vi "HFRR ADV v01.vi"() -> ()   [LabVIEW 2023] (continued)
1.5095757095675688, 1.5106502499343546, 1.5103432384009872, 1.5104967441676709, 1.5111107672344057, 1.5104967441676709, 1.5103432384009872, 1.5112642730010895, 1.5108037557010383, 1.5103432384009872, 1.5104967441676709, 1.5106502499343546, 1.5106502499343546, 1.5108037557010383, 1.5111107672344057, 1.5095757095675688, 1.5097292153342525, 1.5111107672344057, 1.5104967441676709, 1.5138738710347124, 1.5138738710347124, 1.5124923191345592, 1.5115712845344569, 1.510957261467722, 1.509422203800885, 1.5108037557010383, 1.5104967441676709, 1.5101897326343034, 1.5104967441676709, 1.5101897326343034, 1.5101897326343034, 1.5103432384009872, 1.5101897326343034, 1.5104967441676709, 1.5101897326343034, 1.5108037557010383, 1.5106502499343546, 1.5098827211009362, 1.5112642730010895, 1.5098827211009362, 1.510957261467722, 1.5104967441676709, 1.5101897326343034, 1.5101897326343034, 1.5103432384009872, 1.5108037557010383, 1.5097292153342525, 1.5111107672344057, 1.5108037557010383, 1.5104967441676709, 1.5112642730010895, 1.5103432384009872, 1.5097292153342525, 1.5104967441676709, 1.5106502499343546, 1.5108037557010383, 1.5100362268676197, 1.5106502499343546, 1.5106502499343546, 1.5103432384009872, 1.5097292153342525, 1.5106502499343546, 1.5100362268676197, 1.5111107672344057, 1.5108037557010383, 1.5100362268676197, 1.5101897326343034, 1.5117247903011406, 1.5117247903011406, 1.510957261467722, 1.5100362268676197, 1.510957261467722, 1.5112642730010895, 1.5103432384009872, 1.5112642730010895, 1.5098827211009362, 1.5112642730010895, 1.510957261467722, 1.5106502499343546, 1.5123388133678755, 1.5123388133678755, 1.5103432384009872, 1.5101897326343034, 1.5101897326343034, 1.5104967441676709, 1.5097292153342525, 1.5111107672344057, 1.5108037557010383, 1.5126458249012429, 1.5117247903011406, 1.5100362268676197, 1.5106502499343546, 1.5098827211009362, 1.5104967441676709, 1.5098827211009362, 1.5106502499343546, 1.5115712845344569, 1.5108037557010383, 1.5112642730010895, 1.5100362268676197, 1.5112642730010895, 1.5104967441676709, 1.5098827211009362, 1.5091151922675177, 1.5112642730010895, 1.5103432384009872, 1.514641399868131, 1.5154089287015495, 1.5117247903011406, 1.5111107672344057, 1.5101897326343034, 1.5098827211009362, 1.5106502499343546, 1.5106502499343546, 1.5106502499343546, 1.5106502499343546, 1.5104967441676709, 1.5112642730010895, 1.5103432384009872, 1.5108037557010383, 1.5106502499343546, 1.5097292153342525, 1.510957261467722, 1.5112642730010895, 1.5103432384009872, 1.510957261467722, 1.5112642730010895, 1.5111107672344057, 1.5106502499343546, 1.5097292153342525, 1.5101897326343034, 1.5097292153342525, 1.5114177787677732, 1.5100362268676197, 1.5103432384009872, 1.5114177787677732, 1.5104967441676709, 1.5112642730010895, 1.5108037557010383, 1.509422203800885, 1.5108037557010383, 1.510957261467722, 1.5108037557010383, 1.5108037557010383, 1.5106502499343546, 1.5108037557010383, 1.510957261467722, 1.5117247903011406, 1.5092686980342014, 1.5098827211009362, 1.5108037557010383, 1.5104967441676709, 1.510957261467722, 1.5111107672344057, 1.5114177787677732, 1.5114177787677732, 1.5114177787677732, 1.5100362268676197, 1.509422203800885, 1.5114177787677732, 1.5106502499343546, 1.5100362268676197, 1.5108037557010383, 1.5103432384009872, 1.5108037557010383, 1.510957261467722, 1.5101897326343034, 1.5103432384009872, 1.5098827211009362, 1.5114177787677732, 1.5108037557010383, 1.5104967441676709, 1.510957261467722, 1.5101897326343034, 1.5111107672344057, 1.5106502499343546, 1.5103432384009872, 1.5108037557010383, 1.5095757095675688, 1.5106502499343546, 1.5103432384009872, 1.5104967441676709, 1.5111107672344057, 1.5104967441676709, 1.5103432384009872, 1.5112642730010895, 1.5108037557010383, 1.5103432384009872, 1.5104967441676709, 1.5106502499343546, 1.5106502499343546, 1.5108037557010383, 1.5111107672344057, 1.5095757095675688, 1.5097292153342525, 1.5111107672344057, 1.5104967441676709, 1.5138738710347124, 1.5138738710347124, 1.5124923191345592, 1.5115712845344569, 1.510957261467722, 1.509422203800885, 1.5108037557010383, 1.5104967441676709, 1.5101897326343034, 1.5104967441676709, 1.5101897326343034, 1.5101897326343034, 1.5103432384009872, 1.5101897326343034, 1.5104967441676709, 1.5101897326343034, 1.5108037557010383, 1.5106502499343546, 1.5098827211009362, 1.5112642730010895, 1.5098827211009362, 1.510957261467722, 1.5104967441676709, 1.5101897326343034, 1.5101897326343034, 1.5103432384009872, 1.5108037557010383, 1.5097292153342525, 1.5111107672344057, 1.5108037557010383, 1.5104967441676709, 1.5112642730010895, 1.5103432384009872, 1.5097292153342525, 1.5104967441676709, 1.5106502499343546, 1.5108037557010383, 1.5100362268676197, 1.5106502499343546, 1.5106502499343546, 1.5103432384009872, 1.5097292153342525, 1.5106502499343546, 1.5100362268676197, 1.5111107672344057, 1.5108037557010383, 1.5100362268676197, 1.5101897326343034, 1.5117247903011406, 1.5117247903011406, 1.510957261467722, 1.5100362268676197, 1.510957261467722, 1.5112642730010895, 1.5103432384009872, 1.5112642730010895, 1.5098827211009362, 1.5112642730010895, 1.510957261467722, 1.5106502499343546, 1.5123388133678755, 1.5123388133678755, 1.5103432384009872, 1.5101897326343034, 1.5101897326343034, 1.5104967441676709, 1.5097292153342525, 1.5111107672344057, 1.5108037557010383, 1.5126458249012429, 1.5117247903011406, 1.5100362268676197, 1.5106502499343546, 1.5098827211009362, 1.5104967441676709, 1.5098827211009362, 1.5106502499343546, 1.5115712845344569, 1.5108037557010383, 1.5112642730010895, 1.5100362268676197, 1.5112642730010895, 1.5104967441676709, 1.5098827211009362, 1.5091151922675177, 1.5112642730010895, 1.5103432384009872, 1.514641399868131, 1.5154089287015495, 1.5117247903011406, 1.5111107672344057, 1.5101897326343034, 1.5098827211009362, 1.5106502499343546, 1.5106502499343546, 1.5106502499343546, 1.5106502499343546, 1.5104967441676709, 1.5112642730010895, 1.5103432384009872, 1.5108037557010383, 1.5106502499343546, 1.5097292153342525, 1.510957261467722, 1.5112642730010895, 1.5103432384009872, 1.510957261467722, 1.5112642730010895, 1.5111107672344057, 1.5106502499343546, 1.5097292153342525, 1.5101897326343034, 1.5097292153342525, 1.5114177787677732, 1.5100362268676197, 1.5103432384009872, 1.5114177787677732, 1.5104967441676709, 1.5112642730010895, 1.5108037557010383, 1.509422203800885, 1.5108037557010383, 1.510957261467722, 1.5108037557010383, 1.5108037557010383, 1.5106502499343546, 1.5108037557010383, 1.510957261467722, 1.5117247903011406, 1.5092686980342014, 1.5098827211009362, 1.5108037557010383, 1.5104967441676709, 1.510957261467722, 1.5111107672344057, 1.5114177787677732, 1.5114177787677732, 1.5114177787677732, 1.5100362268676197, 1.509422203800885, 1.5114177787677732, 1.5106502499343546, 1.5100362268676197, 1.5108037557010383, 1.5103432384009872, 1.5108037557010383, 1.510957261467722, 1.5101897326343034, 1.5103432384009872, 1.5098827211009362, 1.5114177787677732, 1.5108037557010383, 1.5104967441676709, 1.510957261467722, 1.5101897326343034, 1.5111107672344057, 1.5106502499343546, 1.5103432384009872, 1.5108037557010383, 1.5095757095675688, 1.5106502499343546, 1.5103432384009872, 1.5104967441676709, 1.5111107672344057, 1.5104967441676709, 1.5103432384009872, 1.5112642730010895, 1.5108037557010383, 1.5103432384009872, 1.5104967441676709, 1.5106502499343546, 1.5106502499343546, 1.5108037557010383, 1.5111107672344057, 1.5095757095675688, 1.5097292153342525, 1.5111107672344057, 1.5104967441676709, 1.5138738710347124, 1.5138738710347124, 1.5124923191345592, 1.5115712845344569, 1.510957261467722, 1.509422203800885, 1.5108037557010383, 1.5104967441676709, 1.5101897326343034, 1.5104967441676709, 1.5101897326343034, 1.5101897326343034, 1.5103432384009872, 1.5101897326343034, 1.5104967441676709, 1.5101897326343034, 1.5108037557010383, 1.5106502499343546, 1.5098827211009362, 1.5112642730010895, 1.5098827211009362, 1.510957261467722, 1.5104967441676709, 1.5101897326343034, 1.5101897326343034, 1.5103432384009872, 1.5108037557010383, 1.5097292153342525, 1.5111107672344057, 1.5108037557010383, 1.5104967441676709, 1.5112642730010895, 1.5103432384009872, 1.5097292153342525, 1.5104967441676709, 1.5106502499343546, 1.5108037557010383, 1.5100362268676197, 1.5106502499343546, 1.5106502499343546, 1.5103432384009872, 1.5097292153342525, 1.5106502499343546, 1.5100362268676197, 1.5111107672344057, 1.5108037557010383, 1.5100362268676197, 1.5101897326343034, 1.5117247903011406, 1.5117247903011406, 1.510957261467722, 1.5100362268676197, 1.510957261467722, 1.5112642730010895, 1.5103432384009872, 1.5112642730010895, 1.5098827211009362, 1.5112642730010895, 1.510957261467722, 1.5106502499343546, 1.5123388133678755, 1.5123388133678755, 1.5103432384009872, 1.5101897326343034, 1.5101897326343034, 1.5104967441676709, 1.5097292153342525, 1.5111107672344057, 1.5108037557010383, 1.5126458249012429, 1.5117247903011406, 1.5100362268676197, 1.5106502499343546, 1.5098827211009362, 1.5104967441676709, 1.5098827211009362, 1.5106502499343546, 1.5115712845344569, 1.5108037557010383, 1.5112642730010895, 1.5100362268676197, 1.5112642730010895, 1.5104967441676709, 1.5098827211009362, 1.5091151922675177, 1.5112642730010895, 1.5103432384009872, 1.514641399868131, 1.5154089287015495, 1.5117247903011406, 1.5111107672344057, 1.5101897326343034, 1.5098827211009362, 1.5106502499343546, 1.5106502499343546, 1.5106502499343546, 1.5106502499343546, 1.5104967441676709, 1.5112642730010895, 1.5103432384009872, 1.5108037557010383, 1.5106502499343546, 1.5097292153342525, 1.510957261467722, 1.5112642730010895, 1.5103432384009872, 1.510957261467722, 1.5112642730010895, 1.5111107672344057, 1.5106502499343546, 1.5097292153342525, 1.5101897326343034, 1.5097292153342525, 1.5114177787677732, 1.5100362268676197, 1.5103432384009872, 1.5114177787677732, 1.5104967441676709, 1.5112642730010895, 1.5108037557010383, 1.509422203800885, 1.5108037557010383, 1.510957261467722, 1.5108037557010383, 1.5108037557010383, 1.5106502499343546, 1.5108037557010383, 1.510957261467722, 1.5117247903011406, 1.5092686980342014, 1.5098827211009362, 1.5108037557010383, 1.5104967441676709, 1.510957261467722, 1.5111107672344057, 1.5114177787677732, 1.5114177787677732, 1.5114177787677732, 1.5100362268676197, 1.509422203800885, 1.5114177787677732, 1.5106502499343546, 1.5100362268676197, 1.5108037557010383, 1.5103432384009872, 1.5108037557010383, 1.510957261467722, 1.5101897326343034, 1.5103432384009872, 1.5098827211009362, 1.5114177787677732, 1.5108037557010383, 1.5104967441676709, 1.510957261467722, 1.5101897326343034, 1.5111107672344057, 1.5106502499343546, 1.5103432384009872, 1.5108037557010383, 1.5095757095675688, 1.5106502499343546, 1.5103432384009872, 1.5104967441676709, 1.5111107672344057, 1.5104967441676709, 1.5103432384009872, 1.5112642730010895, 1.5108037557010383, 1.5103432384009872, 1.5104967441676709, 1.5106502499343546, 1.5106502499343546, 1.5108037557010383, 1.5111107672344057, 1.5095757095675688, 1.5097292153342525, 1.5111107672344057, 1.5104967441676709, 1.5138738710347124, 1.5138738710347124, 1.5124923191345592, 1.5115712845344569, 1.510957261467722, 1.509422203800885, 1.5108037557010383, 1.5104967441676709, 1.5101897326343034, 1.5104967441676709, 1.5101897326343034, 1.5101897326343034, 1.5103432384009872, 1.5101897326343034, 1.5104967441676709, 1.5101897326343034, 1.5108037557010383, 1.5106502499343546, 1.5098827211009362, 1.5112642730010895, 1.5098827211009362, 1.510957261467722, 1.5104967441676709, 1.5101897326343034, 1.5101897326343034, 1.5103432384009872, 1.5108037557010383, 1.5097292153342525, 1.5111107672344057, 1.5108037557010383, 1.5104967441676709, 1.5112642730010895, 1.5103432384009872, 1.5097292153342525, 1.5104967441676709, 1.5106502499343546, 1.5108037557010383, 1.5100362268676197, 1.5106502499343546, 1.5106502499343546, 1.5103432384009872, 1.5097292153342525, 1.5106502499343546, 1.5100362268676197, 1.5111107672344057, 1.5108037557010383, 1.5100362268676197, 1.5101897326343034, 1.5117247903011406, 1.5117247903011406, 1.510957261467722, 1.5100362268676197, 1.510957261467722, 1.5112642730010895, 1.5103432384009872, 1.5112642730010895, 1.5098827211009362, 1.5112642730010895, 1.510957261467722, 1.5106502499343546, 1.5123388133678755, 1.5123388133678755, 1.5103432384009872, 1.5101897326343034, 1.5101897326343034, 1.5104967441676709, 1.5097292153342525, 1.5111107672344057, 1.5108037557010383, 1.5126458249012429, 1.5117247903011406, 1.5100362268676197, 1.5106502499343546, 1.5098827211009362, 1.5104967441676709, 1.5098827211009362, 1.5106502499343546, 1.5115712845344569, 1.5108037557010383, 1.5112642730010895, 1.5100362268676197, 1.5112642730010895, 1.5104967441676709, 1.5098827211009362, 1.5091151922675177, 1.5112642730010895, 1.5103432384009872, 1.514641399868131, 1.5154089287015495, 1.5117247903011406, 1.5111107672344057, 1.5101897326343034, 1.5098827211009362, 1.5106502499343546, 1.5106502499343546, 1.5106502499343546, 1.5106502499343546, 1.5104967441676709, 1.5112642730010895, 1.5103432384009872, 1.5108037557010383, 1.5106502499343546, 1.5097292153342525, 1.510957261467722, 1.5112642730010895, 1.5103432384009872, 1.510957261467722, 1.5112642730010895, 1.5111107672344057, 1.5106502499343546, 1.5097292153342525, 1.5101897326343034, 1.5097292153342525, 1.5114177787677732, 1.5100362268676197, 1.5103432384009872, 1.5114177787677732, 1.5104967441676709, 1.5112642730010895, 1.5108037557010383, 1.509422203800885, 1.5108037557010383, 1.510957261467722, 1.5108037557010383, 1.5108037557010383, 1.5106502499343546, 1.5108037557010383, 1.510957261467722, 1.5117247903011406, 1.5092686980342014, 1.5098827211009362, 1.5108037557010383, 1.5104967441676709, 1.510957261467722, 1.5111107672344057, 1.5114177787677732, 1.5114177787677732, 1.5114177787677732, 1.5100362268676197, 1.509422203800885, 1.5114177787677732, 1.5106502499343546, 1.5100362268676197, 1.5108037557010383, 1.5103432384009872, 1.5108037557010383, 1.510957261467722, 1.5101897326343034, 1.5103432384009872, 1.5098827211009362, 1.5114177787677732, 1.5108037557010383, 1.5104967441676709, 1.510957261467722, 1.5101897326343034, 1.5111107672344057, 1.5106502499343546, 1.5103432384009872, 1.5108037557010383, 1.5095757095675688, 1.5106502499343546, 1.5103432384009872, 1.5104967441676709, 1.5111107672344057, 1.5104967441676709, 1.5103432384009872, 1.5112642730010895, 1.5108037557010383, 1.5103432384009872, 1.5104967441676709, 1.5106502499343546, 1.5106502499343546, 1.5108037557010383, 1.5111107672344057, 1.5095757095675688, 1.5097292153342525, 1.5111107672344057, 1.5104967441676709, 1.5138738710347124, 1.5138738710347124, 1.5124923191345592, 1.5115712845344569, 1.510957261467722, 1.509422203800885, 1.5108037557010383, 1.5104967441676709, 1.5101897326343034, 1.5104967441676709, 1.5101897326343034, 1.5101897326343034, 1.5103432384009872, 1.5101897326343034, 1.5104967441676709, 1.5101897326343034, 1.5108037557010383, 1.5106502499343546, 1.5098827211009362, 1.5112642730010895, 1.5098827211009362, 1.510957261467722, 1.5104967441676709, 1.5101897326343034, 1.5101897326343034, 1.5103432384009872, 1.5108037557010383, 1.5097292153342525, 1.5111107672344057, 1.5108037557010383, 1.5104967441676709, 1.5112642730010895, 1.5103432384009872, 1.5097292153342525, 1.5104967441676709, 1.5106502499343546, 1.5108037557010383, 1.5100362268676197, 1.5106502499343546, 1.5106502499343546, 1.5103432384009872, 1.5097292153342525, 1.5106502499343546, 1.5100362268676197, 1.5111107672344057, 1.5108037557010383, 1.5100362268676197, 1.5101897326343034, 1.5117247903011406, 1.5117247903011406, 1.510957261467722, 1.5100362268676197, 1.510957261467722, 1.5112642730010895, 1.5103432384009872, 1.5112642730010895, 1.5098827211009362, 1.5112642730010895, 1.510957261467722, 1.5106502499343546, 1.5123388133678755, 1.5123388133678755, 1.5103432384009872, 1.5101897326343034, 1.5101897326343034, 1.5104967441676709, 1.5097292153342525, 1.5111107672344057, 1.5108037557010383, 1.5126458249012429, 1.5117247903011406, 1.5100362268676197, 1.5106502499343546, 1.5098827211009362, 1.5104967441676709, 1.5098827211009362, 1.5106502499343546, 1.5115712845344569, 1.5108037557010383, 1.5112642730010895, 1.5100362268676197, 1.5112642730010895, 1.5104967441676709, 1.5098827211009362, 1.5091151922675177, 1.5112642730010895, 1.5103432384009872, 1.514641399868131, 1.5154089287015495, 1.5117247903011406, 1.5111107672344057, 1.5101897326343034, 1.5098827211009362, 1.5106502499343546, 1.5106502499343546, 1.5106502499343546, 1.5106502499343546, 1.5104967441676709, 1.5112642730010895, 1.5103432384009872, 1.5108037557010383, 1.5106502499343546, 1.5097292153342525, 1.510957261467722, 1.5112642730010895, 1.5103432384009872, 1.510957261467722, 1.5112642730010895, 1.5111107672344057, 1.5106502499343546, 1.5097292153342525, 1.5101897326343034, 1.5097292153342525, 1.5114177787677732, 1.5100362268676197, 1.5103432384009872, 1.5114177787677732, 1.5104967441676709, 1.5112642730010895, 1.5108037557010383, 1.509422203800885, 1.5108037557010383, 1.510957261467722, 1.5108037557010383, 1.5108037557010383, 1.5106502499343546, 1.5108037557010383, 1.510957261467722, 1.5117247903011406, 1.5092686980342014, 1.5098827211009362, 1.5108037557010383, 1.5104967441676709, 1.510957261467722, 1.5111107672344057, 1.5114177787677732, 1.5114177787677732, 1.5114177787677732, 1.5100362268676197, 1.509422203800885, 1.5114177787677732, 1.5106502499343546, 1.5100362268676197, 1.5108037557010383, 1.5103432384009872, 1.5108037557010383, 1.510957261467722, 1.5101897326343034, 1.5103432384009872, 1.5098827211009362, 1.5114177787677732, 1.5108037557010383, 1.5104967441676709, 1.510957261467722, 1.5101897326343034, 1.5111107672344057, 1.5106502499343546, 1.5103432384009872, 1.5108037557010383, 1.5095757095675688, 1.5106502499343546, 1.5103432384009872, 1.5104967441676709, 1.5111107672344057, 1.5104967441676709, 1.5103432384009872, 1.5112642730010895, 1.5108037557010383, 1.5103432384009872, 1.5104967441676709, 1.5106502499343546, 1.5106502499343546, 1.5108037557010383, 1.5111107672344057, 1.5095757095675688, 1.5097292153342525, 1.5111107672344057, 1.5104967441676709, 1.5138738710347124, 1.5138738710347124, 1.5124923191345592, 1.5115712845344569, 1.510957261467722, 1.509422203800885, 1.5108037557010383, 1.5104967441676709, 1.5101897326343034, 1.5104967441676709, 1.5101897326343034, 1.5101897326343034, 1.5103432384009872, 1.5101897326343034, 1.5104967441676709, 1.5101897326343034, 1.5108037557010383, 1.5106502499343546, 1.5098827211009362, 1.5112642730010895, 1.5098827211009362, 1.510957261467722, 1.5104967441676709, 1.5101897326343034, 1.5101897326343034, 1.5103432384009872, 1.5108037557010383, 1.5097292153342525, 1.5111107672344057, 1.5108037557010383, 1.5104967441676709, 1.5112642730010895, 1.5103432384009872, 1.5097292153342525, 1.5104967441676709, 1.5106502499343546, 1.5108037557010383, 1.5100362268676197, 1.5106502499343546, 1.5106502499343546, 1.5103432384009872, 1.5097292153342525, 1.5106502499343546, 1.5100362268676197, 1.5111107672344057, 1.5108037557010383, 1.5100362268676197, 1.5101897326343034, 1.5117247903011406, 1.5117247903011406, 1.510957261467722, 1.5100362268676197, 1.510957261467722, 1.5112642730010895, 1.5103432384009872, 1.5112642730010895, 1.5098827211009362, 1.5112642730010895, 1.510957261467722, 1.5106502499343546, 1.5123388133678755, 1.5123388133678755, 1.5103432384009872, 1.5101897326343034, 1.5101897326343034, 1.5104967441676709, 1.5097292153342525, 1.5111107672344057, 1.5108037557010383, 1.5126458249012429, 1.5117247903011406, 1.5100362268676197, 1.5106502499343546, 1.5098827211009362, 1.5104967441676709, 1.5098827211009362, 1.5106502499343546, 1.5115712845344569, 1.5108037557010383, 1.5112642730010895, 1.5100362268676197, 1.5112642730010895, 1.5104967441676709, 1.5098827211009362, 1.5091151922675177, 1.5112642730010895, 1.5103432384009872, 1.514641399868131, 1.5154089287015495, 1.5117247903011406, 1.5111107672344057, 1.5101897326343034, 1.5098827211009362, 1.5106502499343546, 1.5106502499343546, 1.5106502499343546, 1.5106502499343546, 1.5104967441676709, 1.5112642730010895, 1.5103432384009872, 1.5108037557010383, 1.5106502499343546, 1.5097292153342525, 1.510957261467722, 1.5112642730010895, 1.5103432384009872, 1.510957261467722, 1.5112642730010895, 1.5111107672344057, 1.5106502499343546, 1.5097292153342525, 1.5101897326343034, 1.5097292153342525, 1.5114177787677732, 1.5100362268676197, 1.5103432384009872, 1.5114177787677732, 1.5104967441676709, 1.5112642730010895, 1.5108037557010383, 1.509422203800885, 1.5108037557010383, 1.510957261467722, 1.5108037557010383, 1.5108037557010383, 1.5106502499343546, 1.5108037557010383, 1.510957261467722, 1.5117247903011406, 1.5092686980342014, 1.5098827211009362, 1.5108037557010383, 1.5104967441676709, 1.510957261467722, 1.5111107672344057, 1.5114177787677732, 1.5114177787677732, 1.5114177787677732, 1.5100362268676197, 1.509422203800885, 1.5114177787677732, 1.5106502499343546, 1.5100362268676197, 1.5108037557010383, 1.5103432384009872, 1.5108037557010383, 1.510957261467722, 1.5101897326343034, 1.5103432384009872, 1.5098827211009362, 1.5114177787677732, 1.5108037557010383, 1.5104967441676709, 1.510957261467722, 1.5101897326343034, 1.5111107672344057, 1.5106502499343546, 1.5103432384009872, 1.5108037557010383, 1.5095757095675688, 1.5106502499343546, 1.5103432384009872, 1.5104967441676709, 1.5111107672344057, 1.5104967441676709, 1.5103432384009872, 1.5112642730010895, 1.5108037557010383, 1.5103432384009872, 1.5104967441676709, 1.5106502499343546, 1.5106502499343546, 1.5108037557010383, 1.5111107672344057, 1.5095757095675688, 1.5097292153342525, 1.5111107672344057, 1.5104967441676709, 1.5138738710347124, 1.5138738710347124, 1.5124923191345592, 1.5115712845344569, 1.510957261467722, 1.509422203800885, 1.5108037557010383, 1.5104967441676709, 1.5101897326343034, 1.5104967441676709, 1.5101897326343034, 1.5101897326343034, 1.5103432384009872, 1.5101897326343034, 1.5104967441676709, 1.5101897326343034, 1.5108037557010383, 1.5106502499343546, 1.5098827211009362, 1.5112642730010895, 1.5098827211009362, 1.510957261467722, 1.5104967441676709, 1.5101897326343034, 1.5101897326343034, 1.5103432384009872, 1.5108037557010383, 1.5097292153342525, 1.5111107672344057, 1.5108037557010383, 1.5104967441676709, 1.5112642730010895, 1.5103432384009872, 1.5097292153342525, 1.5104967441676709, 1.5106502499343546, 1.5108037557010383, 1.5100362268676197, 1.5106502499343546, 1.5106502499343546, 1.5103432384009872, 1.5097292153342525, 1.5106502499343546, 1.5100362268676197, 1.5111107672344057, 1.5108037557010383, 1.5100362268676197, 1.5101897326343034, 1.5117247903011406, 1.5117247903011406, 1.510957261467722, 1.5100362268676197, 1.510957261467722, 1.5112642730010895, 1.5103432384009872]
  out "Numeric":i32=178
  out "Flag":dbl format="%.2f"
  in  "Tab Control 3":enum32{"RMS", "LIVE"}(tab)
  out "array w/ subset deleted":dbl[](array[numeric])
  out "REMARKS":string="@WINDUCOM : RECIPROCATORY TEST RIG    DEFINITON FILE       \r  Sample ID :- , Load :-  2.00 N , Remarks :- , Date :- 05/11/2016, 06:04\r"
  out "Time 2":dbl=0.0004
  in  "reinit":bool=TRUE
  in  "Remarks : 2":string
  out "Err Count":i32
  out "PID-out":dbl
  out "Rate":dbl=2500.0 caption="Rate (Hz)" min=100.0 max=10000.0 step=1.0
  out "COUNT":i32
  out "FRICVALZ":dbl
  out "Sensor mean 3":dbl
  out "Sensor mean":dbl(slide) min=0.0 max=5.0 step=0.001 scale=0.0..5.0
  out "Sensor mean 2":dbl
  in  "ao0":errorcluster
  out "String 2":string
  out "clk":dbl min=0.0 max=999999999.0 step=0.25 format="%.2f"
  out "spm":string
  out "stp":dbl=0.25 min=0.25 max=60.0 step=0.25 format="%.2f"
  # "Data points"
  # "Data points"
  # "erfds"
  # "HFRR adv"
  # "HFRR adv"
  # "Test Setup"
  # "SAMPLE INFO"
  # "Hz"
  # "mm"
  # "N"
  # "%RH"
  # "min"
  # "°C"
  # "left"
  # "Data points"
  # "Captured if Stroke is +-0.5 of 1mm"
  # "Stroke calibration Procedure: \n1. Insert step 1 in between pushrod and stud and correct the offeset        value  of high pricision laser displacement sensor and the software value.\n2. Insert step 2 (of 0.5mm) and press the capture button to enter\nthe readings in the table shown below\n3. Follow the procedure 3 times and capture the values in  the table.\n4. Press Calculate button to read the error in the gain value."
  # "Calibration assembly image"
  # "ISO : WS1.4"
  # "Reference Fluid Information"
  # "Note:\nMake sure to place all images in the folder \"C:\\WinDucom\\im\" before clicking on \"Import Image.\""
  # "LAB-IQ-NXT\\ WO 2464 \\ v02 \\ DECEMBER 2025"
  # "NOTE:\nPlace all the images in the path \"C:\\WinDucom\\im\" before clicking on Import Image"
  # "Wear Scar Measurements"
  # "Reference Fluid Information"
  # "Graph :"
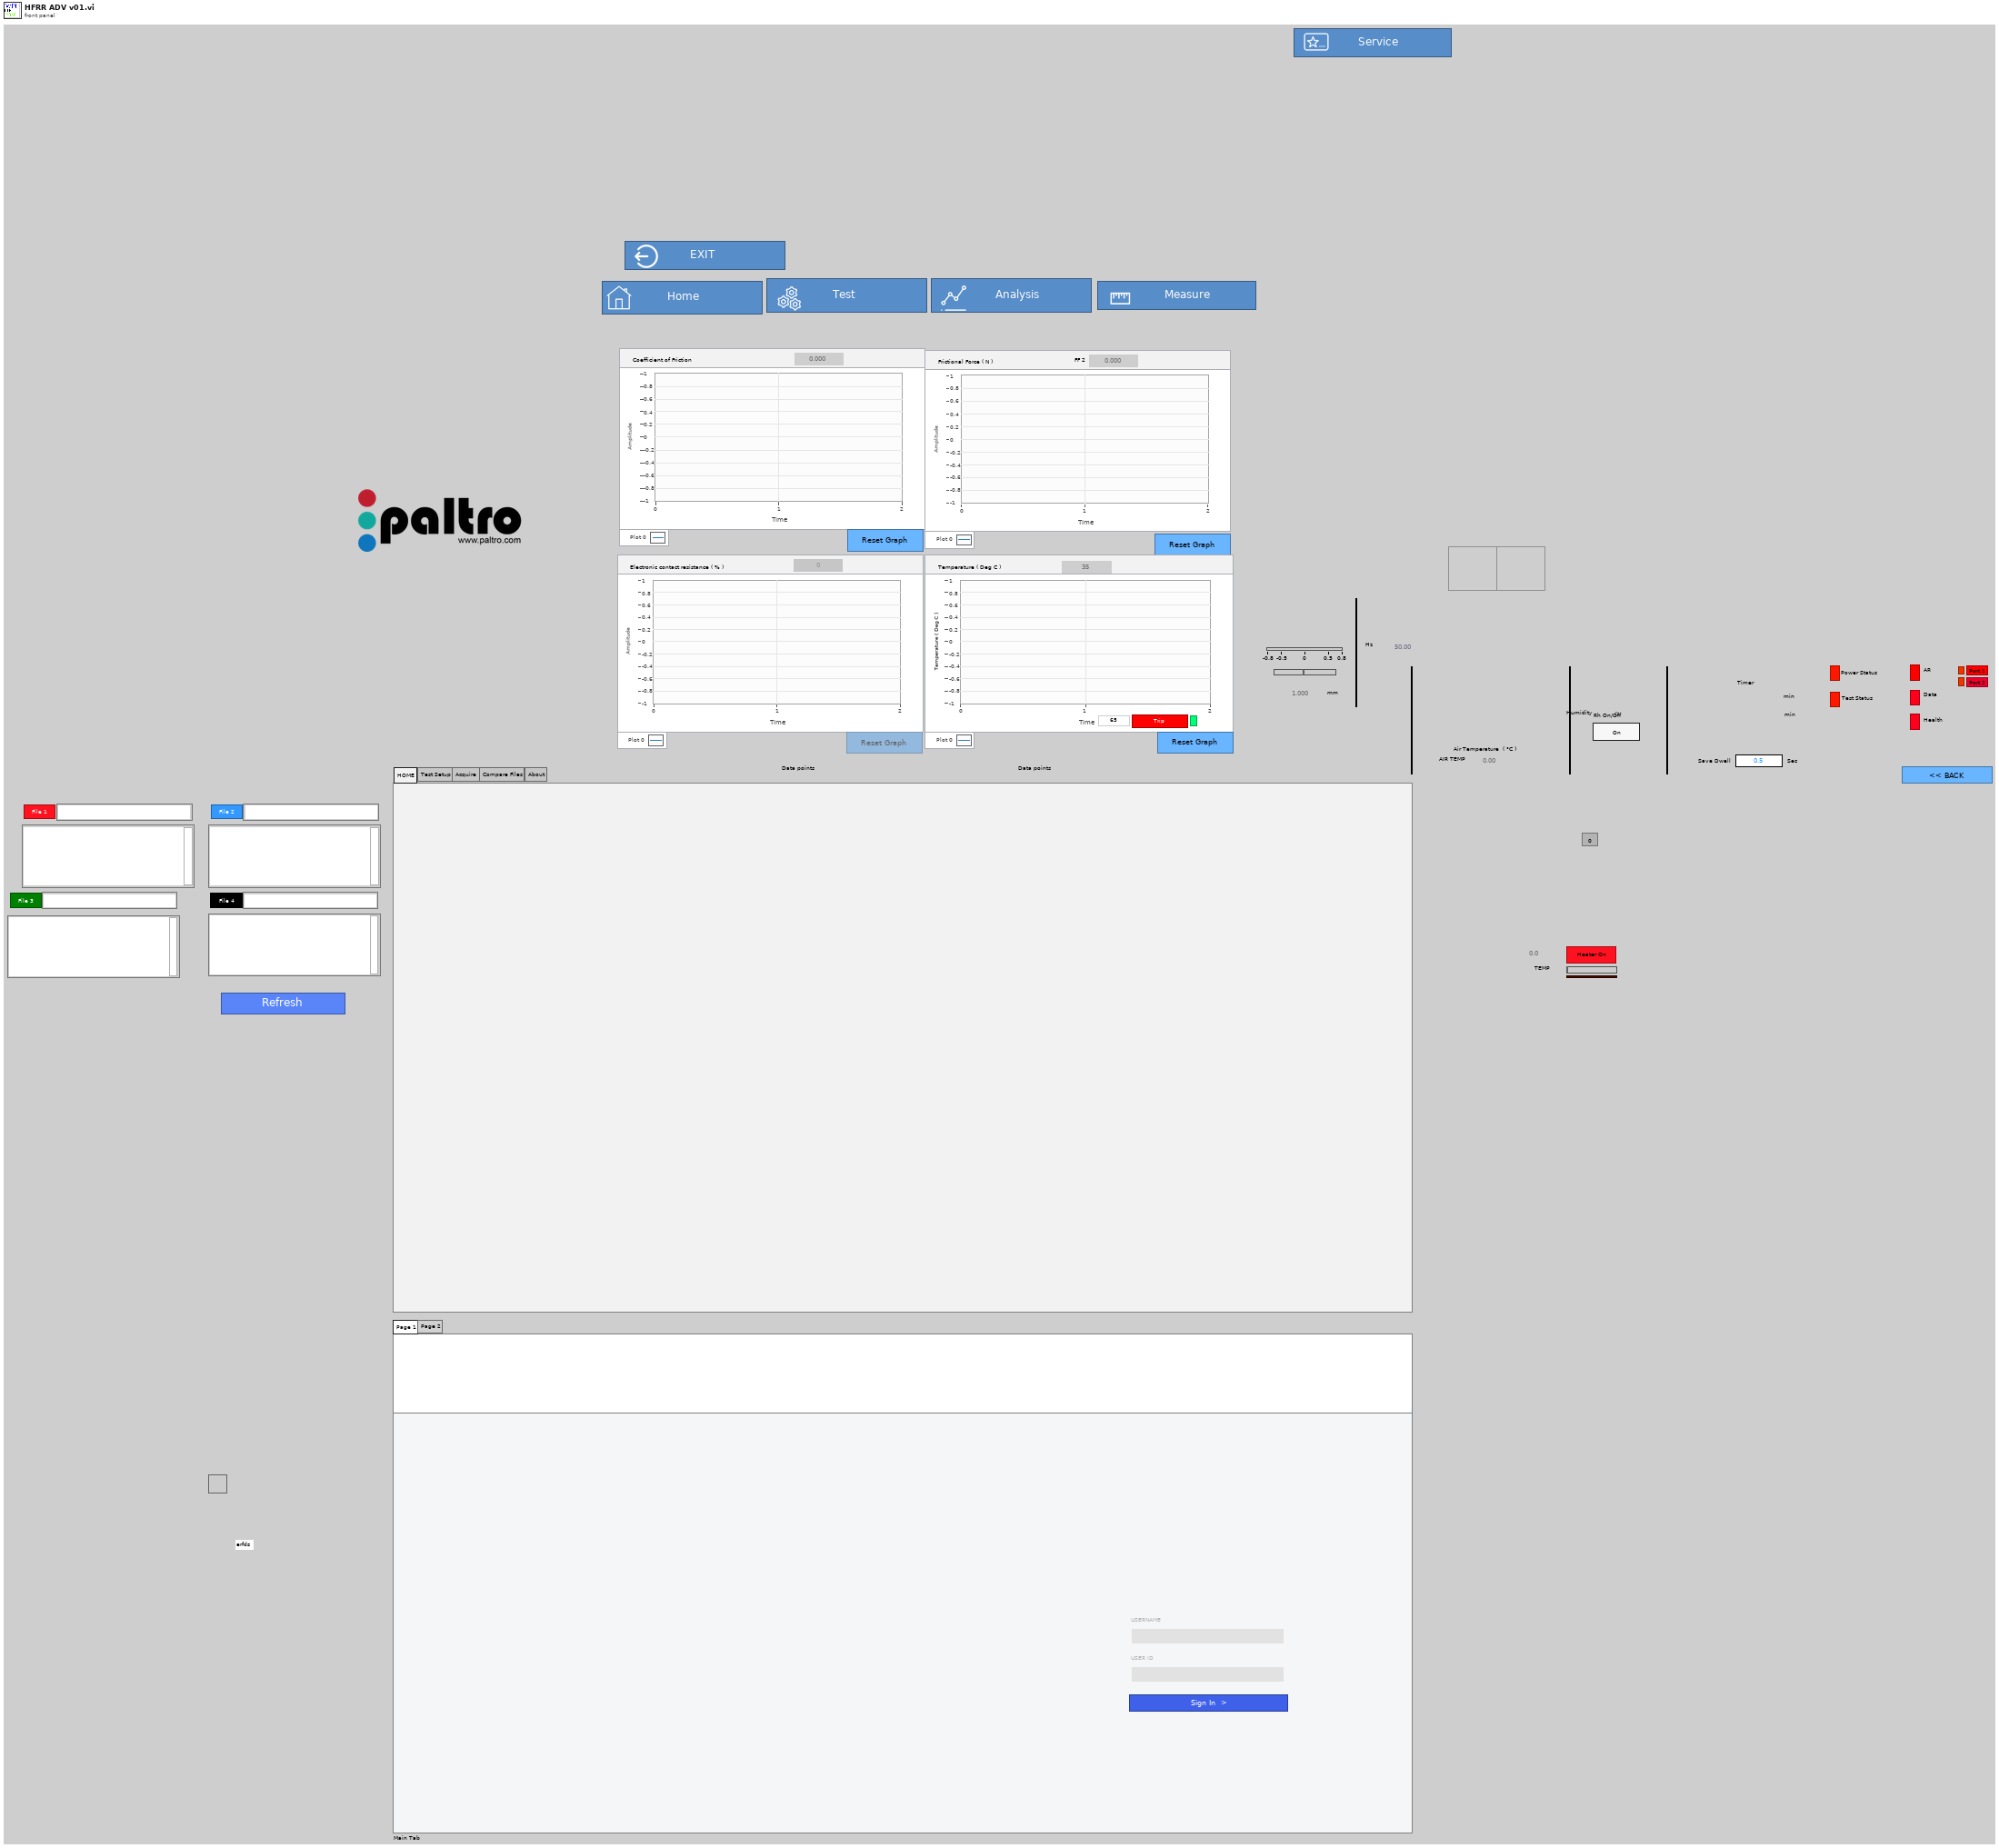
[diagram p1: front panel]
types:
  T1 = enum32{"HOME", "Test Setup", "Acquire", "Compare Files", "About", "Advance", "Mooha"}
  T2 = enum16{"ASTM D6079", "ISO 12156", "CEC F-096-A-06", "Custom"}
  T3 = enum32{"Freqz control", "Low Speed Analog Inputs & Digital IOs", "Temperature Tuning", "Voltage LVDT raw", "High Speed Analog Inputs - Displacement & Friction", "LVDT Calibration", "Sericve", "Friction Force Calibration", "Bytes At Port", "Loadcell Board"}
  T4 = cluster{"proportional gain (Kc)":dbl, "integral time (Ti, min)":dbl, "derivative time (Td, min)":dbl}
  T5 = typedef "imagedata.ctl" = cluster{"image type":i32, "image depth":i32, "image":u8[], "mask":u8[], "colors":u32[], "Rectangle":cluster{"left":i16, "top":i16, "right":i16, "bottom":i16}}
  T6 = enum32{"HOME", "Test Setup", "Acquire", "Compare Files", "Print Report", "About", "Advance", "Mooha"}
  T7 = enum32{"Coefficient Of Friction", "Air Temperature", "Humidity", "Stroke", "Sample Temperature", "Electrical Contact Resistance", "Frequency", "Air Temp vs Rh"}
  T8 = enum32{"Stroke Data", "Temperature Calibration", "Friction Force Raw Data"}
  T9 = cluster{"Proportional Gain (Kc)":dbl, "Integral Time (Ti, min)":dbl, "Derivative Time (Td, min)":dbl}
  T10 = enum32{"   ACQUIRE     ", "   COMPARE   FILES ", "     ABOUT        "}
  T11 = enum32{"ACQUIRE", "COMPARE FILES", "PRINT REPORT", "ABOUT"}
  T12 = enum16{"deny read/write", "deny write-only", "deny none"}
  T13 = typedef "NI_ReportGenerationCore.lvlib/HTML Report Image Alignment.ctl" = enum16{"(default)", "LEFT", "RIGHT", "TOP", "TEXTTOP", "MIDDLE", "ABSMIDDLE", "BASELINE", "BOTTOM", "ABSBOTTOM"}
  T14 = enum16{"open", "replace", "create", "open or create", "replace or create", "replace or create with confirmation"}
  T15 = enum16{"open", "open or create", "create or replace", "create", "open (read only)"}
  T16 = cluster{"Mode":enum16{"RTU", "ASCII"}, "Slave Address":u8}
diagram:
  # "C:\\LAB-IQ-NXT\\calibrate WO 2391.dc"
  # "[CH1]    - FF\n[CH2]   - TEMPERATURE\n[CH3]    - Humidity\n[CH4]    - AIR TEMP\n[CH5]\\- Visa Uno\n[CH6] \\- Visa Due\n[CH7]  \\- file path\n[CH8]   - Displacement Gain\n[CHA]   - Stroke Gain\n[CHB]   - Stroke PID Gain\n[CHC]   -Language Selection\n[CHD]   -Power +\n[CHE]   -Power_\n[CHF]   -Heater\n[CHG]   -Humidity Wet\n[CHH]   -Humidity Dry\n[CHI]   -Integral Time \n[CHIJ   -Air intercept\n[CHI]   -Temp Intercept"
  n1 = flat-sequence {
    tunnel: ["ao0"] -> w5
    tunnel: w5 -> [w104]
    tunnel: [w102] -> w4
    tunnel: [w104] -> w3
    tunnel: [w106] -> w16
    tunnel: [w107] -> w47
    tunnel: w4 -> [w107]
    tunnel: w3 -> [w106]
    frame #0 {
      w50 = FALSE ("Upld AR 2")
      # "password file"
      n2 = Current VI's Path() -> (path=w63:path)
      n3 = Strip Path(path=w63) -> (stripped path=w56:path)  [unwired: 1 out]
      n4 = Path To String(path=w56) -> (string=w58:string)
      n5 = Search/Split String(string=w58, search string/char (-)=".exe") -> (match + rest of string=w60:string)  [unwired: 1 in, 2 out]
      n6 = Match True/False String(2:".vi" ("false string"), 3:".exe" ("true string"), 4:w60) -> (0:w57:bool)  [unwired: 1 out]
      n7 = case shown="True" w57 {
        tunnel: w56 -> [w80 w82]
        tunnel: [w80 w81] -> w54
        frame False {
        }
        frame True {
          n8 = Strip Path(path=w82) -> (stripped path=w81:path)  [unwired: 1 out]
        }
      }
      n9 = Path To String(path=w54) -> (string=→"Gain path":string)
      n10 = List Folder(path=path "C:/Windows" ("directory path"), pattern="*.txt") -> (filenames=w70:string[])  [unwired: 2 in, 3 out]
      n11 = Search 1D Array(1D array=w70, element="wndcm_pw_stdED hfrr.txt") -> (index of element=w73:i32)  [unwired: 1 in]
      n12 = local write "Com flag"(u32 0 ("Com flag")) -> ()
      n13 = Equal?(x=w73, y=-1) -> (x = y?=w68:bool)
      n14 = case shown="True" w68 {
        frame False {
        }
        frame True {
          n15 = String To Byte Array(string="123\n") -> (unsigned byte array=w88:u8[])
          n16 = Array Size(array=w88) -> (size(s)=w87:i32)
          n17 = for {
            N: w87 -> [_]
            tunnel: w88 -> [w101]
            tunnel: [w98] -> w90 mode=indexing
            tunnel: w87 -> [w93]
            i -> [w91]
            n18 = Index Array(array=w101, index=w91) -> (element=w100:u8)
            n19 = Decrement(x=w93) -> (x-1=w94:i32)
            n20 = Equal?(x=w91, y=w94) -> (x = y?=w95:bool)
            n21 = Number To Decimal String(number=w100) -> (decimal integer string=w99:string)  [unwired: 1 in]
            n22 = Select(t="", s=w95, f="\r") -> (s? t:f=w92:string)
            n23 = Concatenate Strings(w99, w92) -> (w98:string)
          }
          n24 = Concatenate Strings(w90) -> (w86:string)
          n25 = local read "file path"() -> (w84:path)
          n26 = call <vilib>:"Write Characters To File.vi"("append to file? (new file:F)"=FALSE, "character string"=w86, "file path (dialog if empty)"=w84) -> ()  [unwired: 2 in, 1 out]
        }
      }
      n27 = local write "refresh flag"(FALSE ("refresh flag")) -> ()
      n28 = local write "Json End Flg"(w50) -> ()
      n29 = local write "Re-Initialise"(TRUE ("Re-Initialise")) -> ()
      n30 = local write "Upld AR 2"(TRUE ("Upld AR 2")) -> ()
      n31 = local write "Json St Flg"(w50) -> ()
      n32 = local write "FLAG 2"(0.0 ("FLAG 2")) -> ()
      n33 = local write "Lan flag"(0.0 ("Lan flag")) -> ()
      n34 = local write "Flag"(0.0 ("Flag")) -> ()
      n35 = local write "clk"(0.0 ("clk")) -> ()
      n36 = local write "COUNT"(0 ("COUNT")) -> ()
      n37 = case shown="True" "STOP" {
        frame False {
        }
        frame True {
          n38 = local write "STOP 3"(TRUE ("STOP")) -> ()
        }
      }
      n39 = local write "conststatus"(0.0 ("rpm value : 2")) -> ()
      "file path" <- path "C:/Windows/wndcm_pw_stdED hfrr.txt" ("file path")
      "FF buffer" <- dbl[] [] ("FF buffer")
    }
    frame #1 {
      n40 = Wait (ms)(milliseconds to wait=u32 1000) -> (millisecond timer value=w102:u32)
    }
    frame #2 {
      n41 = local read "Re-Initialise"() -> (w105:bool)
      n42 = case shown="True" w105 {
        frame False {
        }
        frame True {
          n43 = local write "Re-Initialise"(FALSE ("Re-Initialise")) -> ()
        }
      }
    }
  }
  n44 = while {
    stop <- w113 stop-if-true
    n45 = local read "Image Path"() -> (w111:path)
    n46 = local read "Print 3"() -> (w115:bool)
    n47 = Equal?(x=w111, y=path "") -> (x = y?=w110:bool)
    n48 = Not(x=w110) -> (.not. x?=w109:bool)
    n49 = property on="Print 3" class="Bool (strict)"("Visible"=w109) -> ()  [unwired: 2 in, 2 out]
    n50 = Wait (ms)(milliseconds to wait=u32 20 ("millisecond timer value")) -> ()  [unwired: 1 out]
    n51 = case shown="True" w115 {
      frame False {
        n52 = local write "Rd"(TRUE ("Boolean 7")) -> ()
      }
      frame True {
        n53 = flat-sequence {
          tunnel: [w155] -> w123
          tunnel: [w142] -> w121
          tunnel: [w152] -> w117
          tunnel: w123 -> [w164]
          tunnel: [w164] -> w122
          tunnel: w121 -> [w163]
          tunnel: [w163] -> w120
          tunnel: [w161] -> w119
          tunnel: [w160] -> w118
          tunnel: w117 -> [w160]
          tunnel: w122 -> [w166]
          tunnel: w120 -> [w167]
          tunnel: w119 -> [_]
          tunnel: w118 -> [w165]
          frame #0 {
            n54 = case shown="True" "Rd" {
              frame False {
              }
              frame True {
                n55 = while {
                  tunnel: "abcdefABCDEF" ("string 2") -> [w134]
                  shift-right: [w132] -> w126
                  shift-left: "" -> [w131]
                  i -> [w141]
                  stop <- w140 stop-if-true
                  n56 = Random Number (0-1)() -> (number: 0 to 1=w135:dbl)
                  n57 = Multiply(x=w135, y=62.0) -> (x*y=w137:dbl)
                  n58 = Decrement(x="Length 2") -> (x-1=w130:i16)
                  n59 = To Word Integer(number=w137) -> (16bit integer=w138:i16)
                  n60 = String Subset(string=w134, offset (0)=w138, length (rest)=1 ("length (rest)")) -> (substring=w133:string)
                  n61 = Greater Or Equal?(x=w141, y=w130) -> (x >= y?=w140:bool)
                  n62 = Concatenate Strings(w133, w131) -> (w132:string)
                }
                "String 10" <- w126
                n63 = local write "Rd"(FALSE ("Boolean 7")) -> ()
              }
            }
          }
          frame #1 {
            w153 = "_resized.jpg" ("command line")
            (unwired) ".jpg -resize 320x240 " ("string")
            (unwired) "Choose an Image File" ("prompt")
            # "-resize 1798x425"
            n64 = local read "Image Path"() -> (w147:path)
            n65 = Strip Path(path=w147) -> (stripped path=w142:path, name=w143:string)
            n66 = Match Pattern(string=w143, regular expression=".jpg") -> (before substring=→"before substring 2":string, after substring=→"after substring":string)  [unwired: 1 in, 2 out]
            n67 = Match Pattern(string=w143, regular expression="\\") -> (before substring=w149:string)  [unwired: 1 in, 3 out]
            n68 = Match Pattern(string=w149, regular expression=".jpg") -> (before substring=w148:string)  [unwired: 1 in, 3 out]
            n69 = Concatenate Strings("cmd /c convert " ("string"), w148, ".jpg -resize 320x240  " ("command line"), w148, w153) -> (w156:string)
            n70 = call <vilib>:"System Exec.vi"("run minimized? (F)"=TRUE, "wait until completion? (T)"=TRUE, "working directory"=w142, "command line"=w156) -> ("error out"=w155:errorcluster)  [unwired: 4 in, 3 out]
            "error out 2" <- w155
            n71 = Concatenate Strings(w148, w153) -> (w152:string)
          }
          frame #2 {
            n72 = Wait (ms)(milliseconds to wait=u32 2000 ("millisecond timer value")) -> (millisecond timer value=w161:u32)
          }
          frame #3 {
            n73 = case shown="No Error" w166 {
              tunnel: w167 -> [w170 _]
              tunnel: w165 -> [w168 _]
              frame No Error {
                (unwired) ".jpg" ("string")
                n74 = Path To String(path=w170) -> (string=w174:string)
                n75 = Concatenate Strings(w174, "\\" ("string"), w168) -> (w173:string)
                n76 = String To Path(string=w173) -> (path=w172:path)
                n77 = call <vilib>:"Read JPEG File.vi"("path to JPEG file"=w172) -> ("image data"=w176:T5)  [unwired: 8 in, 2 out]
                "image data" <- w176
                n78 = local write "Print 3"(FALSE ("Print 2")) -> ()
                n79 = call <vilib>:"Draw Flattened Pixmap.vi"("image data"=w176) -> ("new picture"=→"new picture":picture)  [unwired: 8 in]
              }
              frame Error {
              }
            }
          }
        }
      }
    }
    n80 = local read "EXIT"() -> (w113:bool)
  }
  n81 = case shown="True" "Case Constant\n(See Context Help) 7" {
    tunnel: [_ w178] -> w18
    tunnel: w16 -> [_ w177]
    frame False {
    }
    frame True {
      n82 = while {
        tunnel: w177 -> [_]
        tunnel: [w180] -> w178
        tunnel: [w179] -> _
        i -> [w179]
        stop <- w180 stop-if-true
        w196 = u16 10 items=["1.0"=10, "1.5"=15, "2.0"=20] ("stop bits (10: 1 bit)")
        n83 = Wait (ms)(milliseconds to wait=u32 10) -> ()  [unwired: 1 out]
        n84 = call-poly "VISA Configure Serial Port"("VISA resource name"=refnum<visa-resource-name> "ASRL1::INSTR" ("COM PORT"), "timeout (10sec)"=u32 10, "baud rate (9600)"=u32 57600, "data bits (8)"=u16 8, "stop bits (10: 1 bit)"=w196) -> ("VISA resource name out"=w182:refnum<visa-resource-name>, "error out"=w191:errorcluster)  [unwired: 9 in]
        n85 = VISA Read(VISA resource name=w182, byte count=u32 2 ("byte count (0)")) -> (read buffer=w190:string)  [unwired: 1 in, 3 out]
        n86 = String Subset(string=w190, offset (0)=0, length (rest)=2 ("length (rest)")) -> (substring=w189:string)
        n87 = Match Pattern(string=w189, regular expression="<>") -> (offset past match=w186:i32)  [unwired: 1 in, 3 out]
        n88 = Greater Or Equal?(x=w186, y=0) -> (x >= y?=w181:bool)
        n89 = case shown="True" w181 {
          tunnel: w182 -> [_ w200]
          tunnel: w191 -> [_ w199]
          frame False {
          }
          frame True {
            n90 = VISA Read(VISA resource name=w200, byte count=u32 32 ("byte count (0)"), error in (no error)=w199) -> (read buffer=w198:string)  [unwired: 3 out]
            n91 = String Subset(string=w198, offset (0)=0, length (rest)=8 ("length (rest)")) -> (substring=w202:string)
            n92 = String Subset(string=w198, offset (0)=8, length (rest)=8 ("length (rest)")) -> (substring=w203:string)
            n93 = Decimal String To Number(string=w203) -> (number=w210:i32)  [unwired: 2 in, 1 out]
            n94 = Decimal String To Number(string=w202) -> (number=w206:i32)  [unwired: 2 in, 1 out]
            n95 = Divide(x=w210, y=10000) -> ()  [unwired: 1 out]
            n96 = Divide(x=w206, y=1000000) -> ()  [unwired: 1 out]
          }
        }
        n97 = local read "EXIT"() -> (w180:bool)
      }
    }
  }
  n98 = local write "Err Count"(0 ("Err Count")) -> ()
  n99 = local write "FRICVALZ"(0.0 ("FRICVALZ")) -> ()
  n100 = Tick Count (ms)() -> (millisecond timer value=w36:u32)
  n101 = while {
    shift-right: [w227] -> w12
    shift-left: _ -> [w217]
    shift-right: [w226] -> w11
    shift-left: errorcluster {"status"=FALSE, "code"=0, "source"="Init"} ("error out") -> [w219]
    tunnel: [w224] -> w26
    tunnel: [w225] -> _
    tunnel: w16 -> [_]
    i -> [w225]
    stop <- w224 stop-if-true
    n102 = local read "Re-Initialise"() -> (w212:bool)
    n103 = Unbundle(w219) -> ("status"=→"Port 4":bool)  [unwired: 2 out]
    n104 = flat-sequence {
      tunnel: w219 -> [w231]
      tunnel: [w231] -> w215
      frame #0 {
        n105 = Wait (ms)(milliseconds to wait=u32 50) -> ()  [unwired: 1 out]
      }
    }
    n106 = local read "Com Port 2"() -> (w218:refnum<visa-resource-name>)
    n107 = Not Equal?(x=w218, y=w217) -> (x != y?=w216:bool)
    n108 = Or(x=w216, y=w212) -> (x .or. y?=w213:bool)
    n109 = case shown="True" w213 {
      tunnel: [w228 errorcluster {"status"=TRUE, "code"=0, "source"="Init"} ("error out")] -> w214
      tunnel: w215 -> [w228 _]
      frame False {
      }
      frame True {
      }
    }
    n110 = case shown="Error" w214 {
      selector: w214 -> [w234 w388]
      tunnel: [w236 w393] -> w227
      tunnel: [w235 w386] -> w226
      tunnel: w217 -> [w238 w391]
      tunnel: [w237 _] -> _
      frame No Error {
        n111 = stacked-sequence {
          tunnel: w238 -> [w262 _]
          tunnel: w234 -> [w261 _]
          tunnel: [w248 _] -> w237
          tunnel: [w247 _] -> w236
          tunnel: [w246 _] -> w235
          frame #0 {
            n112 = property class="Instr"(reference=w262, error in=w261) -> (reference out=w245:refnum<visa-resource-name>, error out=w260:errorcluster, "Serial Settings:Number of Bytes at Serial Port"=w241:u32)
            "Port 2" <- w241
            n113 = Greater?(x=w241, y=u32 23) -> (0:w243:bool)
            n114 = Not(x=w243) -> ()  [unwired: 1 out]
            n115 = call "Elapsed Time10"("Time Target (s)"=2.0, "Reset"=w243, "Auto Reset"=FALSE) -> ("Time has Elapsed"=→"Port 2a":bool)  [unwired: 9 in, 7 out]
            n116 = case shown="True" w243 {
              tunnel: w245 -> [w277 w302]
              tunnel: w260 -> [w276 w303]
              tunnel: [w276 w305] -> w256
              tunnel: [w277 w304] -> w257
              frame False {
              }
              frame True {
                # "Out as Volts"
                n117 = local read "Residual Due"() -> (w301:string)
                n118 = while {
                  tunnel: [w345] -> w305
                  tunnel: [w344] -> w304
                  tunnel: w303 -> [w343]
                  tunnel: w302 -> [w342]
                  tunnel: [w339] -> _
                  shift-right: [w337] -> w300
                  shift-left: w301 -> [w336]
                  i -> [w339]
                  stop <- w340 stop-if-true
                  n119 = property class="Instr"(reference=w342, error in=w343) -> (reference out=w347:refnum<visa-resource-name>, error out=w346:errorcluster, "Serial Settings:Number of Bytes at Serial Port"=w338:u32)
                  n120 = Greater?(x=w338, y=u32 8) -> (0:w340:bool)
                  n121 = VISA Read(VISA resource name=w347, byte count=w338, error in (no error)=w346) -> (VISA resource name out=w344:refnum<visa-resource-name>, read buffer=w335:string, error out=w345:errorcluster)  [unwired: 1 out]
                  n122 = Concatenate Strings(w336, w335) -> (w337:string)
                }
                n123 = while {
                  shift-right: [w328] -> w284
                  shift-left: w300 -> [w333]
                  tunnel: [w327] -> w296 mode=indexing
                  tunnel: [w326] -> _
                  i -> [w326]
                  stop <- w330 stop-if-true
                  n124 = Match Pattern(string=w333, regular expression="*") -> (after substring=w331:string)  [unwired: 1 in, 3 out]
                  n125 = Match Pattern(string=w331, regular expression="&") -> (before substring=w327:string, after substring=w328:string, offset past match=w329:i32)  [unwired: 1 in, 1 out]
                  n126 = Less Than 0?(x=w329) -> (x < 0?=w330:bool)
                }
                n127 = local write "Residual Due"(w284) -> ()
                n128 = Array Size(array=w296) -> (size(s)=w299:i32)
                n129 = Decrement(x=w299) -> (x-1=w297:i32)
                n130 = Delete From Array(array=w296, length=1, index=w297) -> (array with subset deleted=w295:string[])  [unwired: 1 out]
                n131 = Array Size(array=w295) -> (size(s)=w283:i32)
                n132 = Decrement(x=w283) -> (x-1=w282:i32)
                n133 = while {
                  tunnel: w295 -> [w314] mode=indexing
                  tunnel: w282 -> [w313]
                  tunnel: [w311] -> w290 mode=indexing
                  tunnel: [w310] -> w289 mode=indexing
                  tunnel: [w309] -> w288 mode=indexing
                  tunnel: [w308] -> w287 mode=indexing
                  tunnel: [w307] -> w285 mode=indexing
                  tunnel: [w306] -> _
                  i -> [w306]
                  stop <- w312 stop-if-true
                  w323 = u32 0 ("length (rest)")
                  w322 = ";" ("regular expression")
                  n134 = Match Pattern(string=w314, regular expression=w322) -> (before substring=w315:string, after substring=w316:string)  [unwired: 1 in, 2 out]
                  n135 = Match Pattern(string=w316, regular expression=w322) -> (before substring=w319:string, after substring=w317:string)  [unwired: 1 in, 2 out]
                  n136 = Less Or Equal?(x=w313, y=w306) -> (x <= y?=w312:bool)
                  n137 = Match Pattern(string=w317, regular expression=w322) -> (before substring=w320:string, after substring=w318:string)  [unwired: 1 in, 2 out]
                  n138 = Match Pattern(string=w318, regular expression=w322) -> (before substring=w321:string, after substring=w325:string)  [unwired: 1 in, 2 out]
                  n139 = Decimal String To Number(string=w315, default (0L)=w323) -> (number=w311:u32)  [unwired: 1 in, 1 out]
                  n140 = Decimal String To Number(string=w319, default (0L)=w323) -> (number=w310:u32)  [unwired: 1 in, 1 out]
                  n141 = Decimal String To Number(string=w320, default (0L)=w323) -> (number=w309:u32)  [unwired: 1 in, 1 out]
                  n142 = Decimal String To Number(string=w321, default (0L)=w323) -> (number=w308:u32)  [unwired: 1 in, 1 out]
                  n143 = Decimal String To Number(string=w325, default (0L)=u8 0 ("length (rest)")) -> (number=w307:u8)  [unwired: 1 in, 1 out]
                }
                "Din" <- w285
                n144 = Bundle(w290, w289, w288, w287) -> (w292:cluster{u32[], u32[], u32[], u32[]})  [unwired: 1 in]
                n145 = Divide(x=w292, y=4095 ("length (rest)")) -> (x/y=w294:cluster{dbl[], dbl[], dbl[], dbl[]})
                n146 = Multiply(x=w294, y=sgl 3.32 ("Numeric")) -> (x*y=w286:cluster{dbl[], dbl[], dbl[], dbl[]})
                n147 = Unbundle(w286) -> (→"ECR":dbl[], →"Rtemp":dbl[], →"Air temp":dbl[], →"Ch3 2":dbl[])
              }
            }
            n148 = local read "Due Com"() -> (w249:string[])
            n149 = Delete From Array(array=w249, length=1, index=0) -> (deleted portion=w252:string[], array with subset deleted=w253:string[])
            n150 = local write "Due Com"(w253) -> ()
            n151 = Index Array(array=w252, index=0) -> (element=w250:string)
            n152 = Not Equal?(x=w250, y="") -> (x != y?=w258:bool)
            n153 = case shown="True" w258 {
              tunnel: w257 -> [w264 w269]
              tunnel: [w264 w273] -> w247
              tunnel: w256 -> [w263 w268]
              tunnel: [w263 w271] -> w246
              tunnel: w250 -> [_ w267]
              tunnel: [_ w270] -> _
              frame False {
                # "DATA  WRITE LOOP"
              }
              frame True {
                n154 = Concatenate Strings(w267, "\r\n") -> (w266:string)
                n155 = VISA Write(VISA resource name=w269, write buffer=w266, error in (no error)=w268) -> (VISA resource name out=w273:refnum<visa-resource-name>, return count=w270:u32, error out=w272:errorcluster)
                n156 = flat-sequence {
                  tunnel: w272 -> [w274]
                  tunnel: [w274] -> w271
                  frame #0 {
                    n157 = Wait (ms)(milliseconds to wait=u32 5) -> ()  [unwired: 1 out]
                  }
                }
              }
            }
            n158 = Array Size(array=w249) -> (size(s)=w248:i32)
          }
          frame #1 {
            w356 = 10 ("y")
            w361 = 10 ("y")
            n159 = local read "Rtemp"() -> (w349:dbl[])
            n160 = for {
              tunnel: w349 -> [w373] mode=indexing
              shift-right: [w374] -> w357
              shift-left: dbl[] [] ("temp buf 2") -> [w375]
              n161 = Equal To 0?(x=w373) -> (x = 0?=w377:bool)
              n162 = Build Array (concatenate)(w375, w373) -> (w376:dbl[])
              n163 = Select(t=w375, s=w377, f=w376) -> (s? t:f=w374:dbl[])
            }
            n164 = local read "temp buf"() -> (w358:dbl[])
            n165 = Insert Into Array(array=w357, index=0, new element=w358) -> (w363:dbl[])
            n166 = Array Size(array=w363) -> (size(s)=w362:i32)
            n167 = Greater?(x=w362, y=w361) -> (0:w364:bool)
            n168 = case shown="True" w364 {
              tunnel: w363 -> [w378 w384]
              tunnel: w362 -> [_ w382]
              tunnel: w361 -> [_ w381]
              tunnel: [w378 w379] -> w360
              frame False {
              }
              frame True {
                n169 = Subtract(x=w382, y=w381) -> (x-y=w380:i32)
                n170 = Delete From Array(array=w384, length=w380, index=0) -> (array with subset deleted=w379:dbl[])  [unwired: 1 out]
              }
            }
            "temp buf" <- w360
            n171 = local read "ecr buf"() -> (w350:dbl[])
            n172 = local read "ECR"() -> (w348:dbl[])
            n173 = Insert Into Array(array=w348, index=0, new element=w350) -> (w354:dbl[])
            n174 = Array Size(array=w354) -> (size(s)=w355:i32)
            n175 = Greater?(x=w355, y=w356) -> (0:w353:bool)
            n176 = case shown="True" w353 {
              tunnel: w354 -> [w366 w372]
              tunnel: w355 -> [_ w370]
              tunnel: w356 -> [_ w369]
              tunnel: [w366 w367] -> w351
              frame False {
              }
              frame True {
                n177 = Subtract(x=w370, y=w369) -> (x-y=w368:i32)
                n178 = Delete From Array(array=w372, length=w368, index=0) -> (array with subset deleted=w367:dbl[])  [unwired: 1 out]
              }
            }
            "ecr buf" <- w351
          }
        }
      }
      frame Error {
        w399 = u16 0 items=["None", "XON/XOFF", "RTS/CTS", "XON/XOFF & RTS/CTS", "DTR/DSR", "XON/XOFF & DTR/DSR"] ("flow control (0:none)  2")
        w397 = u16 10 items=["1.0"=10, "1.5"=15, "2.0"=20] ("stop bits 2")
        w395 = u16 0 items=["None", "Odd", "Even", "Mark", "Space"] ("parity 2")
        w396 = u32 10000  # timeout (10sec)
        n179 = VISA Clear(VISA resource name=w391, error in (no error)=w388) -> (VISA resource name out=w390:refnum<visa-resource-name>, error out=w389:errorcluster)
        n180 = VISA Close(VISA resource name=w390, error in (no error)=w389) -> (error out=w392:errorcluster)
        n181 = local read "Com Port 2"() -> (w385:refnum<visa-resource-name>)
        "visa due" <- w385
        n182 = call <vilib>:"Clear Errors.vi"("error in (no error)"=w392) -> ()  [unwired: 5 in, 2 out]
        n183 = call-poly "VISA Configure Serial Port"("VISA resource name"=w385, "timeout (10sec)"=w396, "baud rate (9600)"=u32 250000 ("baud rate  2"), "data bits (8)"=u16 8 ("data bits  2"), "parity (0:none)"=w395, "stop bits (10: 1 bit)"=w397, "flow control (0:none)"=w399) -> ("VISA resource name out"=w400:refnum<visa-resource-name>, "error out"=w401:errorcluster)  [unwired: 7 in]
        n184 = flat-sequence {
          tunnel: w400 -> [w403]
          tunnel: w401 -> [w402]
          tunnel: [w403] -> w393
          tunnel: [w402] -> w386
          frame #0 {
            n185 = Wait (ms)(milliseconds to wait=u32 50) -> ()  [unwired: 1 out]
          }
        }
        "Residual Due" <- ""
        "Port 2 Error" <- w386
      }
    }
    n186 = local read "Port 2a"() -> (w220:bool)
    n187 = local read "Port 4"() -> (w221:bool)
    n188 = Or(x=w221, y=w220) -> (x .or. y?=w223:bool)
    n189 = case shown="True" w223 {
      frame False {
        w232 = FALSE ("Visible")
        n190 = property on="Port 2a" class="Bool (strict)"("Visible"=w232) -> ()  [unwired: 2 in, 2 out]
        n191 = property on="Port 4" class="Bool (strict)"("Visible"=w232) -> ()  [unwired: 2 in, 2 out]
      }
      frame True {
        w233 = TRUE ("Visible")
        n192 = property on="Port 2a" class="Bool (strict)"("Visible"=w233) -> ()  [unwired: 2 in, 2 out]
        n193 = property on="Port 4" class="Bool (strict)"("Visible"=w233) -> ()  [unwired: 2 in, 2 out]
      }
    }
    n194 = local read "EXIT"() -> (w224:bool)
    "Error Due" <- w219
  }
  n195 = while {
    shift-right: [w422] -> w40
    shift-left: _ -> [w410]
    shift-right: [w421] -> w39
    shift-left: errorcluster {"status"=TRUE, "code"=0, "source"="Init"} ("error IO") -> [w412]
    shift-right: [w419] -> _
    shift-left: w36 -> [w420]
    tunnel: w16 -> [_]
    tunnel: [w418] -> w27
    tunnel: [w417] -> _
    i -> [w417]
    stop <- w418 stop-if-true
    n196 = local read "Com Port 1"() -> (w411:refnum<visa-resource-name>)
    n197 = flat-sequence {
      tunnel: [w425] -> w408
      tunnel: w412 -> [w425]
      frame #0 {
        n198 = Wait (ms)(milliseconds to wait=u32 200) -> ()  [unwired: 1 out]
      }
    }
    n199 = local read "Re-Initialise"() -> (w405:bool)
    n200 = Not Equal?(x=w411, y=w410) -> (x != y?=w409:bool)
    n201 = Or(x=w409, y=w405) -> (x .or. y?=w406:bool)
    n202 = Unbundle(w412) -> ("status"=→"Port 3":bool)  [unwired: 2 out]
    n203 = case shown="True" w406 {
      tunnel: [w423 errorcluster {"status"=TRUE, "code"=0, "source"="Init"} ("error out")] -> w407
      tunnel: w408 -> [w423 _]
      frame False {
      }
      frame True {
      }
    }
    n204 = case shown="No Error" w407 {
      selector: w407 -> [w429 w755]
      tunnel: [w434 w760] -> w422
      tunnel: [w433 w752] -> w421
      tunnel: w410 -> [w432 w758]
      tunnel: w420 -> [w431 w757]
      tunnel: [w430 w757] -> w419
      frame No Error {
        n205 = stacked-sequence {
          tunnel: [w444 _ _ _ _ _] -> w434
          tunnel: [w443 _ _ _ _ _] -> w433
          tunnel: w432 -> [w439 _ _ _ _ _]
          tunnel: w429 -> [w438 _ _ _ _ _]
          tunnel: w431 -> [_ w552 _ _ _ _]
          tunnel: [_ w551 _ _ _ _] -> w430
          tunnel: [_ w523 _ _ _ _] -> _
          frame #0 {
            n206 = property class="Instr"(reference=w439, error in=w438) -> (reference out=w441:refnum<visa-resource-name>, error out=w442:errorcluster, "Serial Settings:Number of Bytes at Serial Port"=w435:u32)
            "Sps 3" <- w435
            "Port 1" <- w435
            n207 = Greater?(x=w435, y=u32 5) -> (0:w437:bool)
            n208 = Not(x=w437) -> (.not. x?=→"Port 1a":bool)
            n209 = case shown="True" w437 {
              tunnel: w441 -> [w446 w467]
              tunnel: w442 -> [w445 w468]
              tunnel: [w445 w470] -> w443
              tunnel: [w446 w469] -> w444
              frame False {
              }
              frame True {
                # "Out as Volts"
                n210 = local read "Residual Uno"() -> (w461:string)
                n211 = while {
                  tunnel: [w507] -> w470
                  tunnel: [w506] -> w469
                  tunnel: w468 -> [w505]
                  tunnel: w467 -> [w504]
                  tunnel: [w501] -> _
                  shift-right: [w497] -> w449
                  shift-left: w461 -> [w499]
                  i -> [w501]
                  stop <- w502 stop-if-true
                  n212 = property class="Instr"(reference=w504, error in=w505) -> (reference out=w509:refnum<visa-resource-name>, error out=w508:errorcluster, "Serial Settings:Number of Bytes at Serial Port"=w500:u32)
                  n213 = Greater?(x=w500, y=u32 30) -> (0:w502:bool)
